vi "Detect Barcodes.vi"   [LabVIEW 2020, in "g_ar_toolkit.feature_detection.lvlib" / "BarcodeDetector.lvclass"]
uses:
  BarcodeDetector.lvclass
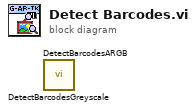
[diagram p0: block diagram]
diagram:
  n1 = call "DetectBarcodesGreyscale.vi"() -> ()  [unwired: 9 in, 3 out]
  n2 = call "DetectBarcodesARGB.vi"() -> ()  [unwired: 9 in, 3 out]
